vi "VTI_Queue_Commands.vi"(1 "VTI Control":T1, 2 "Last status":T1, 3 "20TVTI Queue":refnum<queue>) -> (0 "New Status":T1)   [LabVIEW 2018]
uses:
  S16/VTI-control.ctl
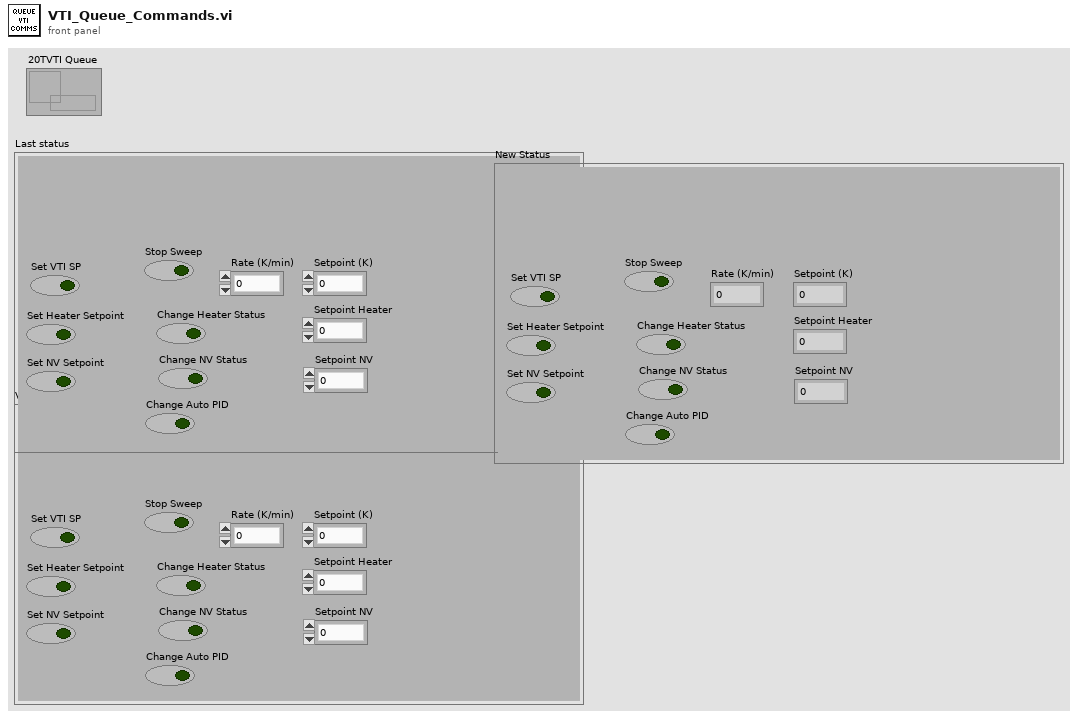
[diagram p1: front panel]
types:
  T1 = typedef "VTI-control.ctl" = cluster{"Set VTI SP":bool, "Change NV Status":bool, "Set NV Setpoint":bool, "Change Heater Status":bool, "Set Heater Setpoint":bool, "Setpoint (K)":dbl, "Rate (K/min)":dbl, "Setpoint Heater":dbl, "Setpoint NV":dbl, "Change Auto PID":bool, "Stop Sweep":bool}
  T2 = cluster{"Set VTI SP":bool, "Change NV Status":bool, "Set NV Setpoint":bool, "Change Heater Status":bool, "Set Heater Setpoint":bool, "Setpoint (K)":bool, "Rate (K/min)":bool, "Setpoint Heater":bool, "Setpoint NV":bool, "Change Auto PID":bool, "Stop Sweep":bool}
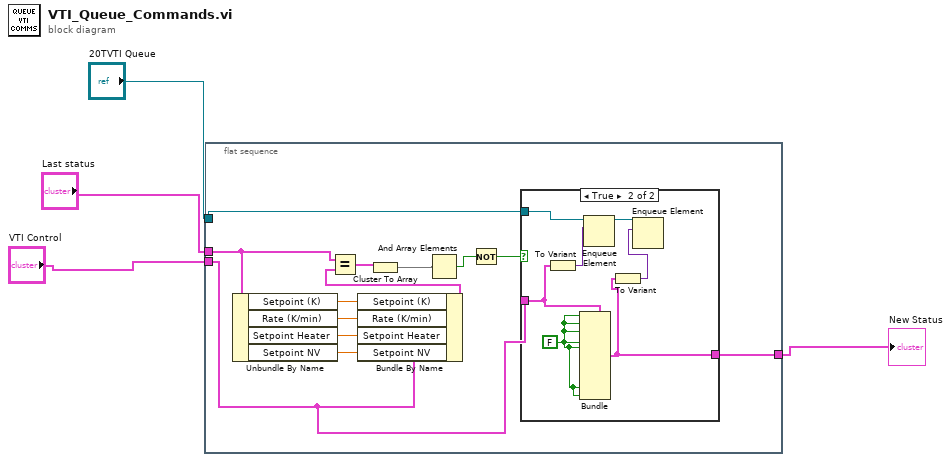
[diagram p0: block diagram]
diagram:
  n1 = flat-sequence {
    tunnel: "20TVTI Queue" -> [w17]
    tunnel: "VTI Control" -> [w11]
    tunnel: "Last status" -> [w9]
    tunnel: [w12] -> w1
    frame #0 {
      n2 = Unbundle By Name(w9) -> ("Setpoint (K)"=w8:dbl, "Rate (K/min)"=w7:dbl, "Setpoint Heater"=w6:dbl, "Setpoint NV"=w5:dbl)
      n3 = Bundle By Name(cluster=w11, "Setpoint (K)"=w8, "Rate (K/min)"=w7, "Setpoint Heater"=w6, "Setpoint NV"=w5) -> (w10:T1)
      n4 = Equal?(x=w9, y=w10) -> (x = y?=w13:T2)
      n5 = Cluster To Array(cluster=w13) -> (array=w16:bool[])
      n6 = And Array Elements(Boolean array=w16) -> (logical AND=w15:bool)
      n7 = Not(x=w15) -> (.not. x?=w14:bool)
      n8 = case shown="True" w14 {
        tunnel: w17 -> [_ w25]
        tunnel: w11 -> [w18 w21]
        tunnel: [w18 w20] -> w12
        frame False {
        }
        frame True {
          w19 = FALSE
          n9 = To Variant(anything=w21) -> (Variant=w24:variant)
          n10 = Bundle(cluster=w21, "Set VTI SP"=w19, "Change NV Status"=w19, "Set NV Setpoint"=w19, "Change Heater Status"=w19, "Set Heater Setpoint"=w19, "Change Auto PID"=w19, "Stop Sweep"=w19) -> (w20:T1)  [unwired: 4 in]
          n11 = Enqueue Element(queue=w25, element=w24) -> (queue out=w23:refnum<queue>)  [unwired: 2 in, 2 out]
          n12 = To Variant(anything=w20) -> (Variant=w22:variant)
          n13 = Enqueue Element(queue=w23, element=w22) -> ()  [unwired: 2 in, 3 out]
        }
      }
    }
  }
  "New Status" <- w1
